vi "Stop.vi"(8 "error in":errorcluster, 11 "Communication in":refnum<class "Communication.lvclass">) -> (0 "error out":errorcluster)   [LabVIEW 2021, in "Communication.lvclass"]
doc: "MIT Licence\nCopyright (c) 2024 David Grollier"
uses:
  Communication.lvclass
  Communication.lvclass/Communication.ctl
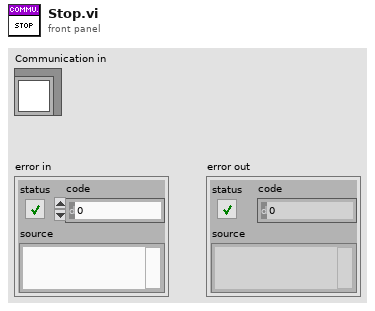
[diagram p1: front panel]
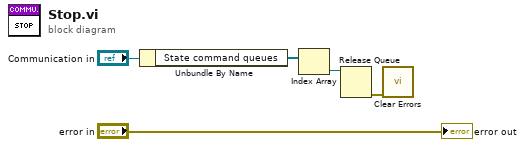
[diagram p0: block diagram]
diagram:
  n1 = Unbundle By Name("Communication in") -> ("State command queues"=w4:refnum<queue>[])
  n2 = Index Array(array=w4) -> (element=w3:refnum<queue>)  [unwired: 1 in]
  n3 = Release Queue(queue=w3) -> (error out=w2:errorcluster)  [unwired: 2 in, 2 out]
  n4 = call <vilib>:"Clear Errors.vi"("error in (no error)"=w2) -> ()  [unwired: 5 in, 2 out]
  "error out" <- "error in"
